vi "PH_Sixpack.StopMotor.vi"(0 "i ref in":refnum<vi>, 1 "axis":i32=-1, 4 "Device Error in":errorcluster, 5 "error in":errorcluster) -> (14 "i ref out":refnum<vi>, 18 "Device Error out":errorcluster, 19 "error out":errorcluster)   [LabVIEW 2014, in "PH_Sixpack.lvlib"]
doc: "This VI acts on the hardware: It stops a movement."
uses:
  PH_Sixpack.lvlib
  instr.lib/Sixpack/Sixpack - Driver.lvlib
  PH_Basics/PH_Stepmotor_BaseClass/PH_Stepmotor_BaseClass.lvlib
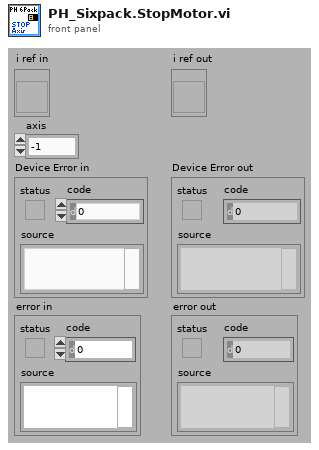
[diagram p1: front panel]
types:
  T1 = cluster{"Boolean array[0]":bool, "Boolean array[1]":bool, "Boolean array[2]":bool, "Boolean array[3]":bool, "Boolean array[4]":bool, "Boolean array[5]":bool}
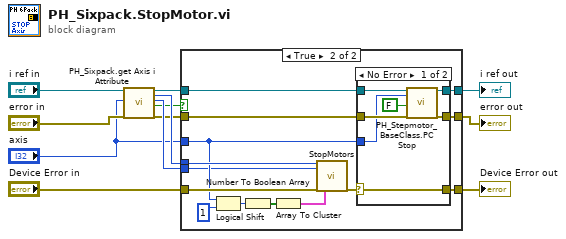
[diagram p0: block diagram]
diagram:
  n1 = call "PH_Sixpack.get Axis i Attribute.vi"("VI in"="i ref in", "Axis"="axis", "error in"="error in") -> ("VI out"=w5:refnum<vi>, "HANDLE"=w10:i32, "SixPack ID(0)"=w9:u16, "Axis found?"=w1:bool, "error out"=w7:errorcluster)  [unwired: 10 in, 2 out]
  n2 = case shown="True" w1 {
    tunnel: w10 -> [_ w29]
    tunnel: w9 -> [_ w16]
    tunnel: "Device Error in" -> [w13 w24]
    tunnel: w7 -> [w14 w23]
    tunnel: [w14 w22] -> w6
    tunnel: w5 -> [w15 w21]
    tunnel: [w15 w20] -> w4
    tunnel: "axis" -> [_ w18]
    tunnel: [w13 w17] -> w2
    frame False {
    }
    frame True {
      n3 = Logical Shift(y=w18, x=1) -> (x << y=w27:i32)
      n4 = Number To Boolean Array(number=w27) -> (Boolean array=w28:bool[])
      n5 = Array To Cluster(array=w28) -> (cluster=w25:T1)
      n6 = call "StopMotors.vi"("handle in"=w29, "UnitAddress(0)"=w16, "error in"=w24, "Motors"=w25) -> ("error out"=w19:errorcluster)  [unwired: 14 in, 1 out]
      n7 = case shown="No Error" w19 {
        selector: w19 -> [w30 w37]
        tunnel: w23 -> [w36 w38]
        tunnel: [w31 w38] -> w22
        tunnel: w21 -> [w35 w39]
        tunnel: [w32 w39] -> w20
        tunnel: w18 -> [w33 _]
        tunnel: [w30 w37] -> w17
        frame No Error {
          n8 = call "PH_Stepmotor_BaseClass.PC Stop.vi"("i ref in"=w35, "axis"=w33, "Stop"=FALSE, "error in (no error)"=w36) -> ("i ref out"=w32:refnum<vi>, "error out"=w31:errorcluster)  [unwired: 14 in]
        }
        frame Error {
        }
      }
    }
  }
  "error out" <- w6
  "i ref out" <- w4
  "Device Error out" <- w2
